vi "filename-manage.vi"(6 "filename pattern":T2, 7 "filename-action":T1=enum."parse", 9 "folder IN":path=path "C:/data/Ultrasound/birdcage/Hg1201/Test", 10 "string IN":string="^(\\s+)(\\d+)_(.*)_(\\d\\d\\d\\d\\d\\d)\\.dat$", 11 "file name IN":string="f027_lsco2_122317.dat") -> (0 "number OUT":dbl=10.0 format="%#_10f", 1 "string OUT":string="^(\\s+)(\\d+)_(.*)_(\\d\\d\\d\\d\\d\\d)\\.dat$", 3 "filename OUT":string)   [LabVIEW 2021]
uses:
  filename-pattern.ctl
  filename-action.ctl
  <vilib>/Utility/libraryn.llb/Check if File or Folder Exists.vi
  <vilib>/regexp/Match Regular Expression.xnode
panel:
  out "offset past match":i32=-1
  out "whole match":string
  out "unique index out":i32
  out "pattern":string="^(\\s+)(\\d+)_(.*)_(\\d\\d\\d\\d\\d\\d)\\.dat$"
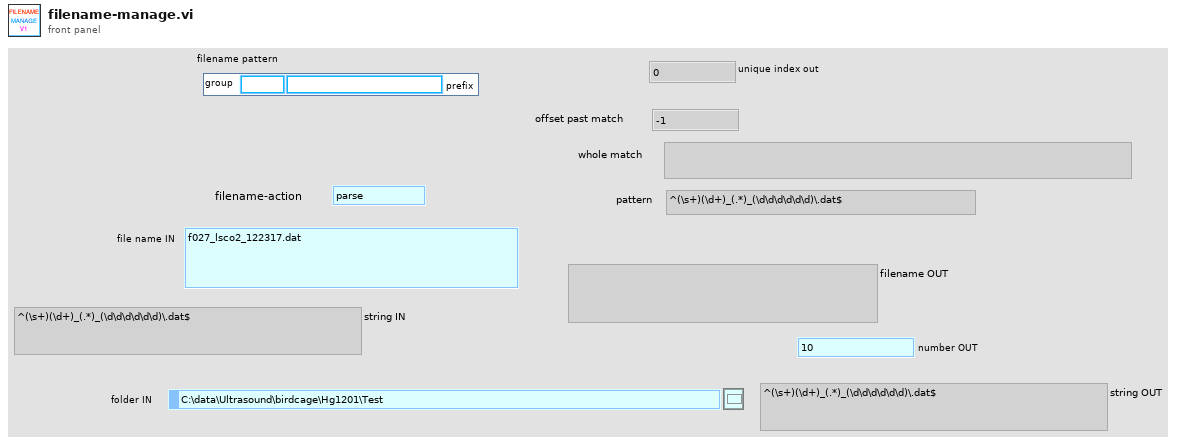
[diagram p1: front panel]
types:
  T1 = typedef "filename-action.ctl" = enum16{"rewrite", "parse", "force pattern", "uniquenum", "get T", "get B", "get ind", "get deg", "get name", "get folder", "get extension", "get basename", "get side", "get setof", "getID", "getIDStock", "remove prefix"}
  T2 = typedef "filename-pattern.ctl" = cluster{"prefix":string, "group":string}
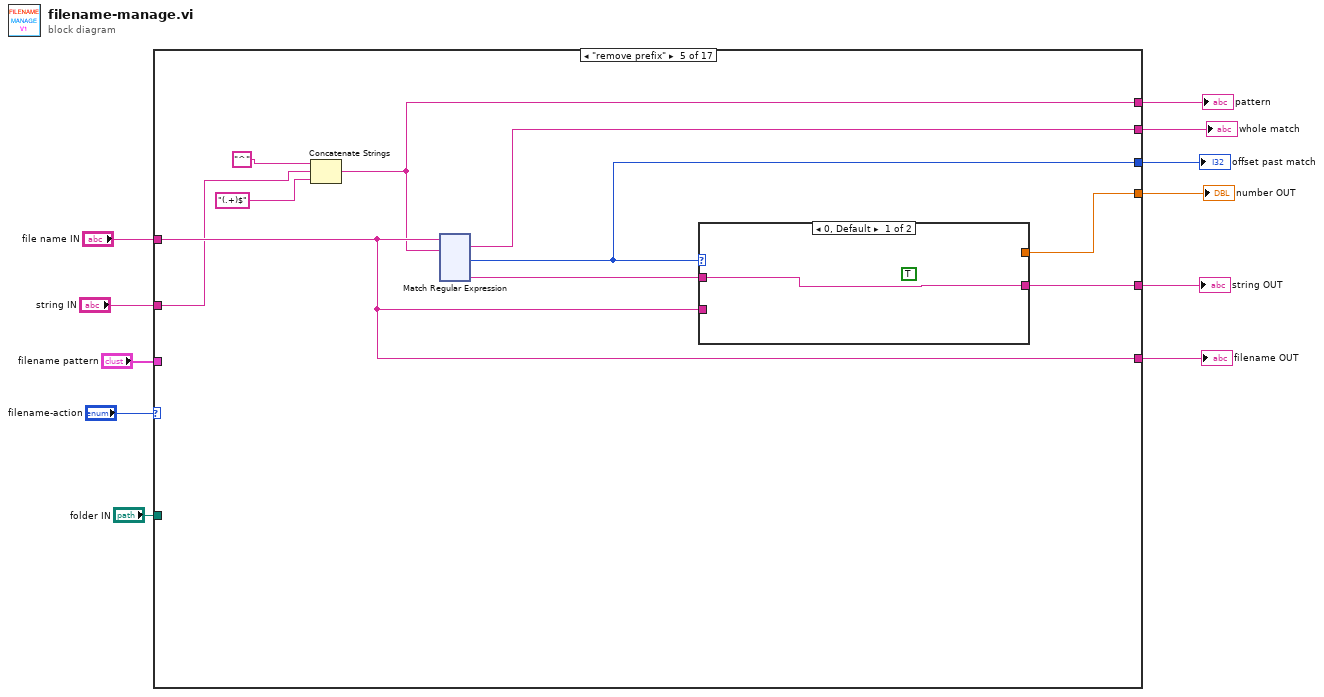
[diagram p0: block diagram]
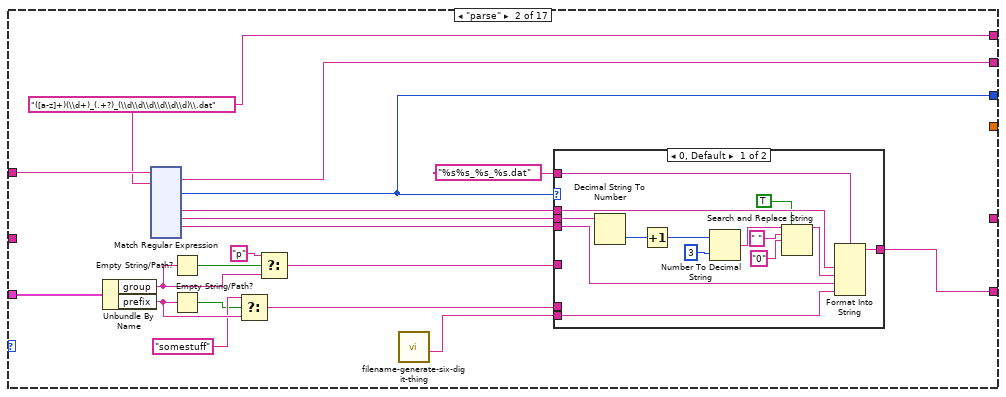
[diagram p3: hidden frame]
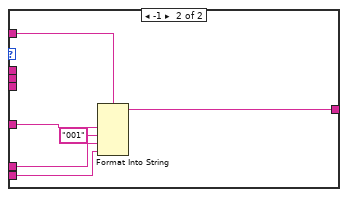
[diagram p4: hidden frame]
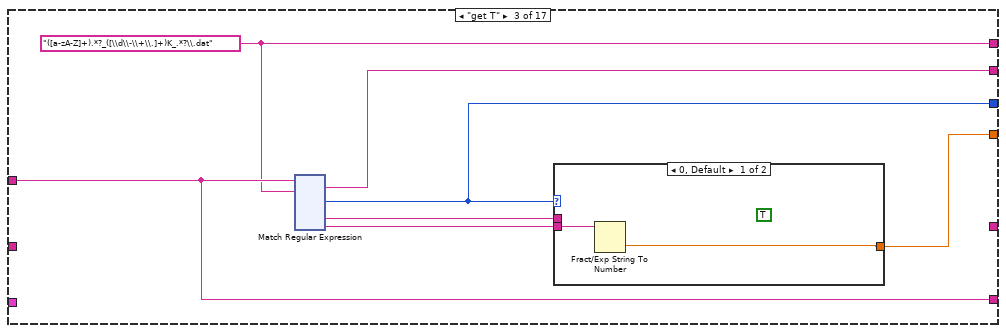
[diagram p5: hidden frame]
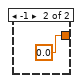
[diagram p6: hidden frame]
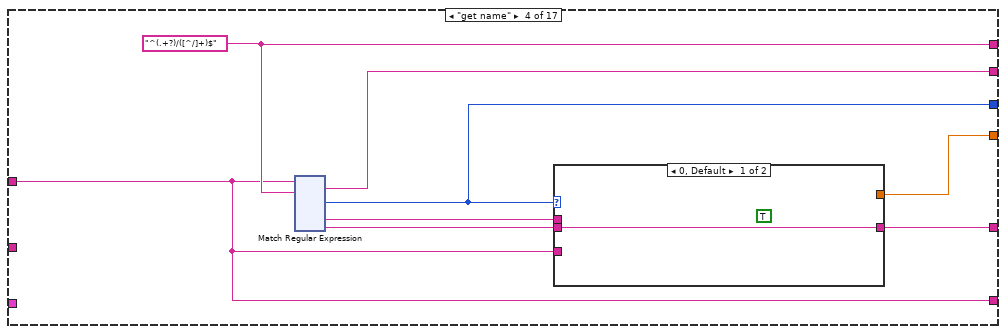
[diagram p7: hidden frame]
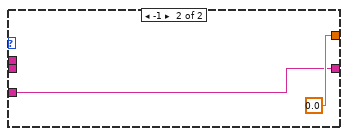
[diagram p8: hidden frame]
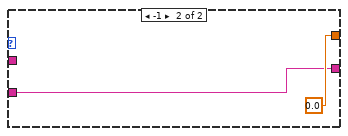
[diagram p9: hidden frame]
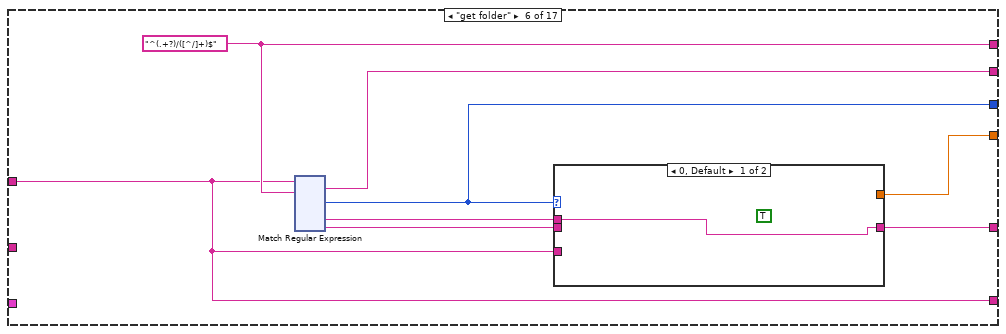
[diagram p10: hidden frame]
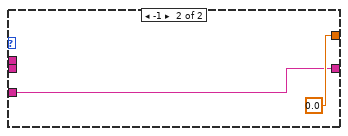
[diagram p11: hidden frame]
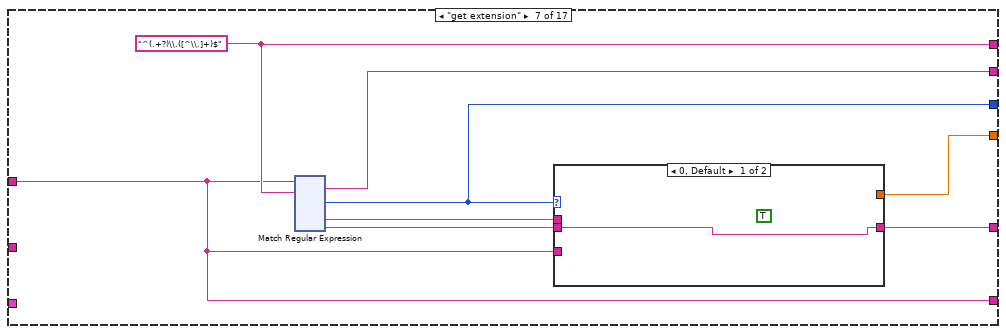
[diagram p12: hidden frame]
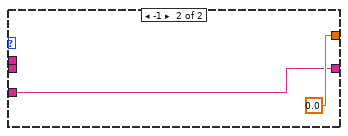
[diagram p13: hidden frame]
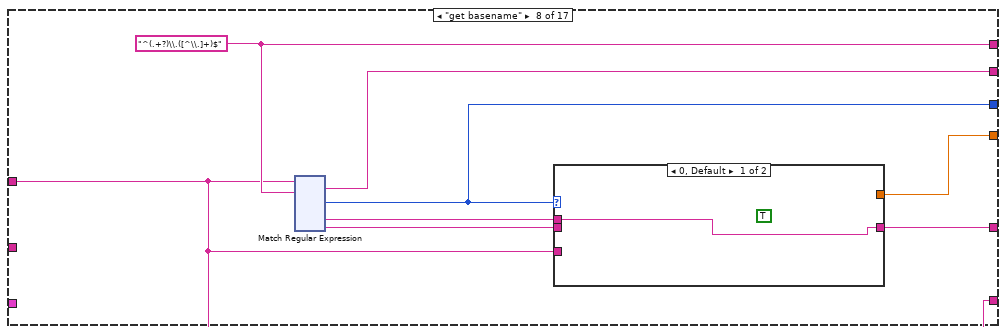
[diagram p14: hidden frame]
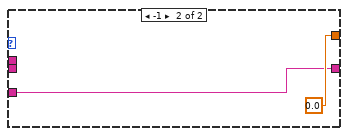
[diagram p15: hidden frame]
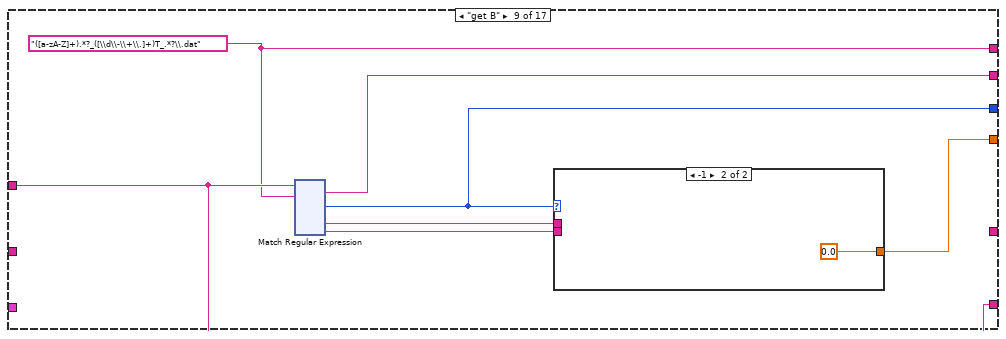
[diagram p16: hidden frame]
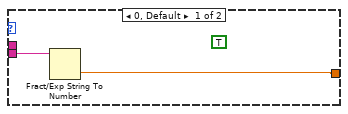
[diagram p17: hidden frame]
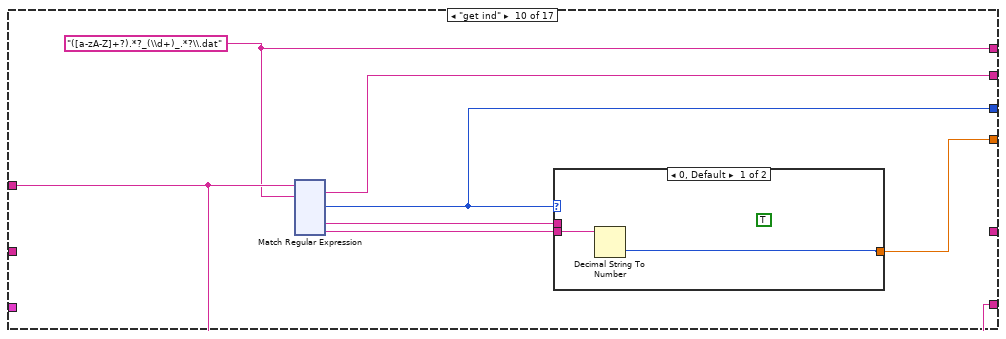
[diagram p18: hidden frame]
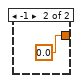
[diagram p19: hidden frame]
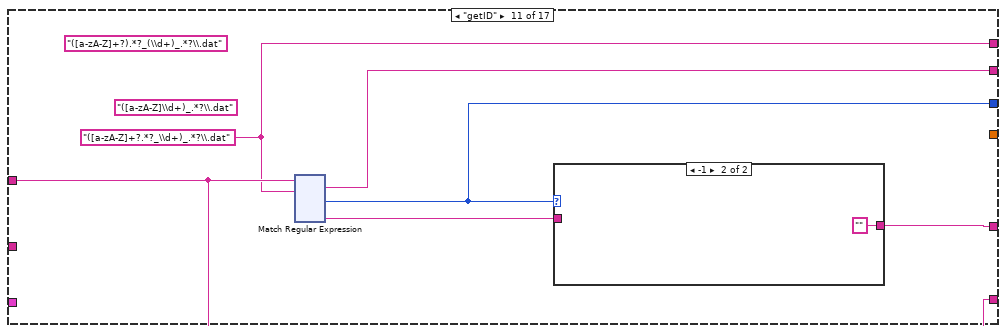
[diagram p20: hidden frame]
diagram:
  n1 = case shown="\"remove prefix\"" "filename-action" {
    tunnel: "file name IN" -> [w12 w31 w178 w304 w439 w567 w698 w829 w964 w1094 w1224 w1347 w1478 w1610 w1740 w1884 w2048]
    tunnel: "filename pattern" -> [_ w30 _ _ _ _ _ _ _ _ _ _ _ _ _ w1883 w2047]
    tunnel: [w12 w20 w178 w304 w439 w567 w698 w829 w964 w1094 w1224 w1347 w1478 w1610 w1740 w1873 w2038] -> w8
    tunnel: "folder IN" -> [_ _ _ _ _ _ _ _ _ _ _ _ _ _ _ _ w2033]
    tunnel: [_ _ w177 w309 w443 w572 w703 w834 w963 w1093 _ _ w1477 w1609 w1739 _ _] -> w6
    tunnel: [_ w13 w176 w308 w442 w571 w702 w833 w962 w1092 w1223 w1351 w1476 w1608 w1738 w1866 w2028] -> w5
    tunnel: [_ w14 w175 w307 w441 w570 w701 w832 w961 w1091 w1222 w1350 w1475 w1607 w1737 w1867 w2027] -> w4
    tunnel: [_ w15 w174 w306 w435 w569 w700 w831 w960 w1090 w1221 w1348 w1474 w1606 w1736 w1868 w2029] -> w3
    tunnel: [_ _ _ w305 w440 w568 w699 w830 _ _ w1220 w1349 _ _ _ _ _] -> w2
    tunnel: "string IN" -> [_ _ _ _ w438 _ _ _ _ _ _ _ _ _ _ _ _]
    frame "rewrite", Default {
    }
    frame "parse" {
      w15 = "([a-z]+)(\\d+)_(.+?)_(\\d\\d\\d\\d\\d\\d)\\.dat" ("format string")
      n2 = Unbundle By Name(w30) -> ("group"=w27:string, "prefix"=w26:string)
      n3 = xnode "Match Regular Expression"("input string"=w31, "regular expression"=w15) -> ("whole match"=w13:string, "offset past match"=w14:i32, "submatch 1"=w18:string, "submatch 2"=w17:string, "submatch 3"=w16:string)  [unwired: 4 in, 4 out]
      n4 = Empty String/Path?(string/path=w27) -> (empty?=w29:bool)
      n5 = Empty String/Path?(string/path=w26) -> (empty?=w24:bool)
      n6 = Select(t="somestuff", s=w24, f=w26) -> (s? t:f=w21:string)
      n7 = Select(t="p", s=w29, f=w27) -> (s? t:f=w22:string)
      n8 = call "filename-generate-six-digit-thing.vi"() -> ("sixdigit"=w19:string)  [unwired: 9 in, 2 out]
      n9 = case shown="0, Default" w14 {
        tunnel: "%s%s_%s_%s.dat" ("format string") -> [w34 w51]
        tunnel: w22 -> [_ w50]
        tunnel: w21 -> [_ w49]
        tunnel: [w44 w48] -> w20
        tunnel: w19 -> [w45 w47]
        tunnel: w18 -> [w43 _]
        tunnel: w17 -> [w42 _]
        tunnel: w16 -> [w33 _]
        frame 0, Default {
          n10 = Decimal String To Number(string=w42) -> (number=w41:i32)  [unwired: 2 in, 1 out]
          n11 = Increment(x=w41) -> (x+1=w40:i32)
          n12 = Number To Decimal String(number=w40, width (-)=i16 3) -> (decimal integer string=w36:string)
          n13 = Search and Replace String(replace all?=TRUE ("replace all? (F)"), input string=w36, search string=" ", replace string="0" ("replace string (\"\")")) -> (result string=w35:string)  [unwired: 4 in, 3 out]
          n14 = Format Into String(format string=w34, w43, w35, w33, w45) -> (resulting string=w44:string)  [unwired: 2 in, 1 out]
        }
        frame -1 {
          n15 = Format Into String(format string=w51, w50, "001" ("input 2"), w49, w47) -> (resulting string=w48:string)  [unwired: 2 in, 1 out]
        }
      }
    }
    frame "get T" {
      w174 = "([a-zA-Z]+).*?_([\\d\\-\\+\\.]+)K_.*?\\.dat" ("format string")
      n16 = xnode "Match Regular Expression"("input string"=w178, "regular expression"=w174) -> ("whole match"=w176:string, "offset past match"=w175:i32, "submatch 1"=w180:string, "submatch 2"=w179:string)  [unwired: 4 in, 3 out]
      n17 = case shown="0, Default" w175 {
        tunnel: [w181 0.0] -> w177
        tunnel: w180 -> [_ _]
        tunnel: w179 -> [w182 _]
        frame 0, Default {
          (unwired) TRUE ("replace all? (F)")
          n18 = Fract/Exp String To Number(string=w182) -> (number=w181:dbl)  [unwired: 3 in, 1 out]
        }
        frame -1 {
        }
      }
    }
    frame "get name" {
      w306 = "^(.+?)/([^/]+)$" ("format string")
      n19 = xnode "Match Regular Expression"("input string"=w304, "regular expression"=w306) -> ("whole match"=w308:string, "offset past match"=w307:i32, "submatch 1"=w311:string, "submatch 2"=w310:string)  [unwired: 4 in, 3 out]
      n20 = case shown="0, Default" w307 {
        tunnel: [_ 0.0] -> w309
        tunnel: w311 -> [_ _]
        tunnel: w310 -> [w312 _]
        tunnel: [w312 w313] -> w305
        tunnel: w304 -> [_ w313]
        frame 0, Default {
          (unwired) TRUE ("replace all? (F)")
        }
        frame -1 {
        }
      }
    }
    frame "remove prefix" {
      n21 = Concatenate Strings("^", w438, "(.+)$" ("format string")) -> (w435:string)
      n22 = xnode "Match Regular Expression"("input string"=w439, "regular expression"=w435) -> ("whole match"=w442:string, "offset past match"=w441:i32, "submatch 1"=w444:string)  [unwired: 4 in, 3 out]
      n23 = case shown="0, Default" w441 {
        tunnel: [_ 0.0] -> w443
        tunnel: w444 -> [w445 _]
        tunnel: [w445 w446] -> w440
        tunnel: w439 -> [_ w446]
        frame 0, Default {
          (unwired) TRUE ("replace all? (F)")
        }
        frame -1 {
        }
      }
    }
    frame "get folder" {
      w569 = "^(.+?)/([^/]+)$" ("format string")
      n24 = xnode "Match Regular Expression"("input string"=w567, "regular expression"=w569) -> ("whole match"=w571:string, "offset past match"=w570:i32, "submatch 1"=w574:string, "submatch 2"=w573:string)  [unwired: 4 in, 3 out]
      n25 = case shown="0, Default" w570 {
        tunnel: [_ 0.0] -> w572
        tunnel: w574 -> [w575 _]
        tunnel: w573 -> [_ _]
        tunnel: [w575 w576] -> w568
        tunnel: w567 -> [_ w576]
        frame 0, Default {
          (unwired) TRUE ("replace all? (F)")
        }
        frame -1 {
        }
      }
    }
    frame "get extension" {
      w700 = "^(.+?)\\.([^\\.]+)$" ("format string")
      n26 = xnode "Match Regular Expression"("input string"=w698, "regular expression"=w700) -> ("whole match"=w702:string, "offset past match"=w701:i32, "submatch 1"=w705:string, "submatch 2"=w704:string)  [unwired: 4 in, 3 out]
      n27 = case shown="0, Default" w701 {
        tunnel: [_ 0.0] -> w703
        tunnel: w705 -> [_ _]
        tunnel: w704 -> [w706 _]
        tunnel: [w706 w707] -> w699
        tunnel: w698 -> [_ w707]
        frame 0, Default {
          (unwired) TRUE ("replace all? (F)")
        }
        frame -1 {
        }
      }
    }
    frame "get basename" {
      w831 = "^(.+?)\\.([^\\.]+)$" ("format string")
      n28 = xnode "Match Regular Expression"("input string"=w829, "regular expression"=w831) -> ("whole match"=w833:string, "offset past match"=w832:i32, "submatch 1"=w836:string, "submatch 2"=w835:string)  [unwired: 4 in, 3 out]
      n29 = case shown="0, Default" w832 {
        tunnel: [_ 0.0] -> w834
        tunnel: w836 -> [w837 _]
        tunnel: w835 -> [_ _]
        tunnel: [w837 w838] -> w830
        tunnel: w829 -> [_ w838]
        frame 0, Default {
          (unwired) TRUE ("replace all? (F)")
        }
        frame -1 {
        }
      }
    }
    frame "get B" {
      w960 = "([a-zA-Z]+).*?_([\\d\\-\\+\\.]+)T_.*?\\.dat" ("format string")
      n30 = xnode "Match Regular Expression"("input string"=w964, "regular expression"=w960) -> ("whole match"=w962:string, "offset past match"=w961:i32, "submatch 1"=w966:string, "submatch 2"=w965:string)  [unwired: 4 in, 3 out]
      n31 = case shown="-1" w961 {
        tunnel: [w967 0.0] -> w963
        tunnel: w966 -> [_ _]
        tunnel: w965 -> [w968 _]
        frame 0, Default {
          (unwired) TRUE ("replace all? (F)")
          n32 = Fract/Exp String To Number(string=w968) -> (number=w967:dbl)  [unwired: 3 in, 1 out]
        }
        frame -1 {
        }
      }
    }
    frame "get ind" {
      w1090 = "([a-zA-Z]+?).*?_(\\d+)_.*?\\.dat" ("format string")
      n33 = xnode "Match Regular Expression"("input string"=w1094, "regular expression"=w1090) -> ("whole match"=w1092:string, "offset past match"=w1091:i32, "submatch 1"=w1096:string, "submatch 2"=w1095:string)  [unwired: 4 in, 3 out]
      n34 = case shown="0, Default" w1091 {
        tunnel: [w1097 0.0] -> w1093
        tunnel: w1096 -> [_ _]
        tunnel: w1095 -> [w1098 _]
        frame 0, Default {
          (unwired) TRUE ("replace all? (F)")
          n35 = Decimal String To Number(string=w1098) -> (number=w1097:i32)  [unwired: 2 in, 1 out]
        }
        frame -1 {
        }
      }
    }
    frame "getID" {
      w1221 = "([a-zA-Z]+?.*?_\\d+)_.*?\\.dat" ("format string")
      (unwired) "([a-zA-Z]\\d+)_.*?\\.dat" ("format string")
      (unwired) "([a-zA-Z]+?).*?_(\\d+)_.*?\\.dat" ("format string")
      n36 = xnode "Match Regular Expression"("input string"=w1224, "regular expression"=w1221) -> ("whole match"=w1223:string, "offset past match"=w1222:i32, "submatch 1"=w1225:string)  [unwired: 4 in, 3 out]
      n37 = case shown="-1" w1222 {
        tunnel: w1225 -> [w1226 _]
        tunnel: [w1226 "" ("submatch 1")] -> w1220
        frame 0, Default {
          (unwired) TRUE ("replace all? (F)")
        }
        frame -1 {
        }
      }
    }
    frame "getIDStock" {
      w1348 = "(IDS\\d+_\\d+_RAW_cal_).*?\\.dat" ("format string")
      (unwired) "([a-zA-Z]+?.*?_\\d+)_.*?\\.dat" ("format string")
      (unwired) "([a-zA-Z]\\d+)_.*?\\.dat" ("format string")
      (unwired) "([a-zA-Z]+?).*?_(\\d+)_.*?\\.dat" ("format string")
      # "IDS0326_210901_RAW_cal_CeCoIn5_4th_055_Rotation.dat"
      n38 = xnode "Match Regular Expression"("input string"=w1347, "regular expression"=w1348) -> ("whole match"=w1351:string, "offset past match"=w1350:i32, "submatch 1"=w1352:string)  [unwired: 4 in, 3 out]
      n39 = case shown="-1" w1350 {
        tunnel: w1352 -> [w1353 _]
        tunnel: [w1353 "" ("submatch 1")] -> w1349
        frame 0, Default {
          (unwired) TRUE ("replace all? (F)")
        }
        frame -1 {
        }
      }
    }
    frame "get side" {
      w1474 = "^([a-zA-Z]+?).*?_(ref|sam)_.*?\\.dat$" ("format string")
      n40 = xnode "Match Regular Expression"("input string"=w1478, "regular expression"=w1474) -> ("whole match"=w1476:string, "offset past match"=w1475:i32, "submatch 1"=w1480:string, "submatch 2"=w1479:string)  [unwired: 4 in, 3 out]
      n41 = case shown="0, Default" w1475 {
        tunnel: [w1481 8000] -> w1477
        tunnel: w1480 -> [_ _]
        tunnel: w1479 -> [w1482 _]
        frame 0, Default {
          n42 = case shown="\"sam\", Default" w1482 {
            tunnel: [8000 4000] -> w1481
            frame "sam", Default {
            }
            frame "ref" {
            }
          }
        }
        frame -1 {
        }
      }
    }
    frame "get setof" {
      w1606 = "[a-zA-Z]+?.*?_(Tdep|Tset|Bdep|Bset)_.*?\\.dat" ("format string")
      # "Tset = 1\nBset = 2"
      n43 = xnode "Match Regular Expression"("input string"=w1610, "regular expression"=w1606) -> ("whole match"=w1608:string, "offset past match"=w1607:i32, "submatch 1"=w1611:string)  [unwired: 4 in, 3 out]
      n44 = case shown="0, Default" w1607 {
        tunnel: [w1613 1.0] -> w1609
        tunnel: w1611 -> [w1612 _]
        frame 0, Default {
          (unwired) TRUE ("replace all? (F)")
          n45 = case shown="\"Tdep\", \"Tset\", Default" w1612 {
            tunnel: [1 2] -> w1613
            frame "Tdep", "Tset", Default {
            }
            frame "Bdep", "Bset" {
            }
          }
        }
        frame -1 {
        }
      }
    }
    frame "get deg" {
      w1736 = "([a-zA-Z]+)_([\\d\\-\\+\\.]+)deg.*?" ("format string")
      (unwired) "([a-zA-Z]+?).*?_(\\d\\d\\d)_.*?\\.dat" ("format string")
      n46 = xnode "Match Regular Expression"("input string"=w1740, "regular expression"=w1736) -> ("whole match"=w1738:string, "offset past match"=w1737:i32, "submatch 1"=w1742:string, "submatch 2"=w1741:string)  [unwired: 4 in, 3 out]
      n47 = case shown="0, Default" w1737 {
        tunnel: [w1743 0.0] -> w1739
        tunnel: w1742 -> [_ _]
        tunnel: w1741 -> [w1744 _]
        frame 0, Default {
          (unwired) TRUE ("replace all? (F)")
          n48 = Decimal String To Number(string=w1744) -> (number=w1743:i32)  [unwired: 2 in, 1 out]
        }
        frame -1 {
        }
      }
    }
    frame "force pattern" {
      w1868 = "([a-z]+)(\\d+)_(.+?)_(\\d\\d\\d\\d\\d\\d)\\.dat" ("format string")
      n49 = Unbundle By Name(w1883) -> ("group"=w1880:string, "prefix"=w1879:string)
      n50 = xnode "Match Regular Expression"("input string"=w1884, "regular expression"=w1868) -> ("whole match"=w1866:string, "offset past match"=w1867:i32, "submatch 1"=w1871:string, "submatch 2"=w1870:string, "submatch 3"=w1869:string)  [unwired: 4 in, 4 out]
      n51 = Empty String/Path?(string/path=w1880) -> (empty?=w1882:bool)
      n52 = Empty String/Path?(string/path=w1879) -> (empty?=w1877:bool)
      n53 = Select(t="somestuff", s=w1877, f=w1879) -> (s? t:f=w1874:string)
      n54 = call "filename-generate-six-digit-thing.vi"() -> ("sixdigit"=w1872:string)  [unwired: 9 in, 2 out]
      n55 = Select(t="p", s=w1882, f=w1880) -> (s? t:f=w1875:string)
      n56 = case shown="0, Default" w1867 {
        tunnel: "%s%s_%s_%s.dat" ("format string") -> [w1888 w1904]
        tunnel: w1875 -> [w1887 w1903]
        tunnel: w1874 -> [w1886 w1902]
        tunnel: [w1897 w1901] -> w1873
        tunnel: w1872 -> [w1898 w1900]
        tunnel: w1871 -> [_ _]
        tunnel: w1870 -> [w1896 _]
        tunnel: w1869 -> [_ _]
        frame 0, Default {
          n57 = Decimal String To Number(string=w1896) -> (number=w1895:i32)  [unwired: 2 in, 1 out]
          n58 = Increment(x=w1895) -> (x+1=w1894:i32)
          n59 = Number To Decimal String(number=w1894, width (-)=i16 3) -> (decimal integer string=w1890:string)
          n60 = Search and Replace String(replace all?=TRUE ("replace all? (F)"), input string=w1890, search string=" ", replace string="0" ("replace string (\"\")")) -> (result string=w1889:string)  [unwired: 4 in, 3 out]
          n61 = Format Into String(format string=w1888, w1887, w1889, w1886, w1898) -> (resulting string=w1897:string)  [unwired: 2 in, 1 out]
        }
        frame -1 {
          n62 = Format Into String(format string=w1904, w1903, "001" ("input 2"), w1902, w1900) -> (resulting string=w1901:string)  [unwired: 2 in, 1 out]
        }
      }
    }
    frame "uniquenum" {
      w2029 = "([a-z]+)(\\d+)_(.+?)_(\\d\\d\\d\\d\\d\\d)\\.dat" ("format string")
      n63 = Unbundle By Name(w2047) -> ("group"=w2044:string, "prefix"=w2043:string)
      n64 = call "file -- 9w path.vi"("sweep folder"=w2033) -> ("9w path"=w2032:path)  [unwired: 10 in]
      n65 = xnode "Match Regular Expression"("input string"=w2048, "regular expression"=w2029) -> ("whole match"=w2028:string, "offset past match"=w2027:i32, "submatch 1"=w2036:string, "submatch 2"=w2035:string, "submatch 3"=w2034:string)  [unwired: 4 in, 4 out]
      n66 = Empty String/Path?(string/path=w2044) -> (empty?=w2046:bool)
      n67 = Empty String/Path?(string/path=w2043) -> (empty?=w2041:bool)
      n68 = Select(t="somestuff", s=w2041, f=w2043) -> (s? t:f=w2039:string)
      n69 = call "filename-generate-six-digit-thing.vi"() -> ("sixdigit"=w2037:string)  [unwired: 9 in, 2 out]
      n70 = Select(t="p", s=w2046, f=w2044) -> (s? t:f=w2031:string)
      n71 = call "file -- get unique increment name.vi"("prefix"=w2031, "9w folder path"=w2032) -> ("unique index out"=w2030:i32)  [unwired: 9 in]
      "unique index out" <- w2030
      n72 = case shown="0, Default" w2027 {
        tunnel: "%s%s_%s_%s.dat" ("format string") -> [w2053 w2066]
        tunnel: w2031 -> [w2052 w2065]
        tunnel: w2039 -> [w2051 w2064]
        tunnel: [w2059 w2063] -> w2038
        tunnel: w2037 -> [w2060 w2062]
        tunnel: w2036 -> [_ _]
        tunnel: w2035 -> [_ _]
        tunnel: w2034 -> [_ _]
        tunnel: w2030 -> [w2050 _]
        frame 0, Default {
          n73 = Number To Decimal String(number=w2050, width (-)=i16 3) -> (decimal integer string=w2055:string)
          n74 = Search and Replace String(replace all?=TRUE ("replace all? (F)"), input string=w2055, search string=" ", replace string="0" ("replace string (\"\")")) -> (result string=w2054:string)  [unwired: 4 in, 3 out]
          n75 = Format Into String(format string=w2053, w2052, w2054, w2051, w2060) -> (resulting string=w2059:string)  [unwired: 2 in, 1 out]
        }
        frame -1 {
          n76 = Format Into String(format string=w2066, w2065, "001" ("input 2"), w2064, w2062) -> (resulting string=w2063:string)  [unwired: 2 in, 1 out]
        }
      }
    }
  }
  "filename OUT" <- w8
  "number OUT" <- w6
  "whole match" <- w5
  "offset past match" <- w4
  "pattern" <- w3
  "string OUT" <- w2
